vi "Handle Error in Client Generation.vi"(8 "error in":errorcluster) -> (0 "error out":errorcluster, 1 "InstrumentStudio Pro < Q4?":bool, 2 "status":T1, 3 "error message":string)   [LabVIEW 2021, in "MeasurementClient Editor.lvlib"]
uses:
  MeasurementClient Editor.lvlib
  Client Creation Status.ctl
  <vilib>/Utility/error.llb/DialogType.ctl
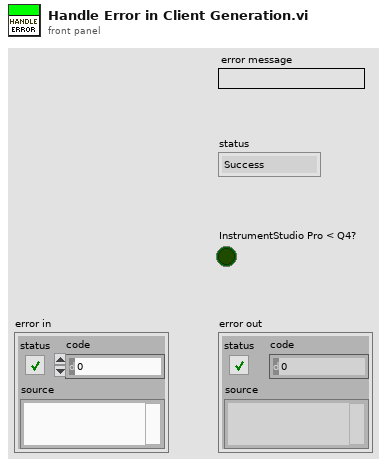
[diagram p1: front panel]
types:
  T1 = typedef "MeasurementClient Editor.lvlib/Client Creation Status.ctl" = enum16{"Success", "Fail"}
  T2 = typedef "DialogType.ctl" = u16
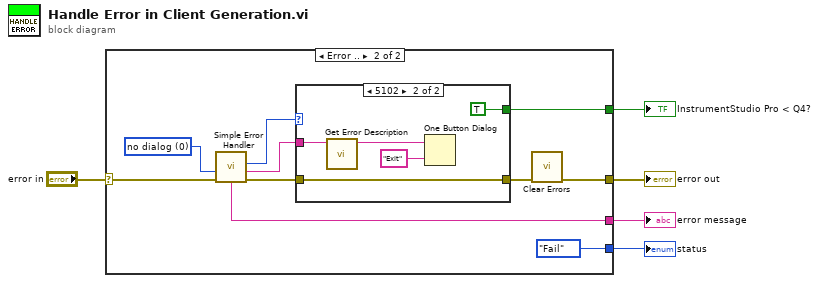
[diagram p0: block diagram]
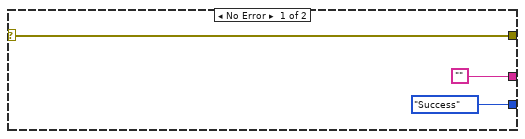
[diagram p2: hidden frame]
diagram:
  n1 = case shown="Error .." "error in" {
    selector: "error in" -> [w8 w18]
    tunnel: [w8 w17] -> w5
    tunnel: ["" w10] -> w3
    tunnel: [_ w12] -> w4
    tunnel: [Client_Creation_Status."Success" ("Enum") Client_Creation_Status."Fail" ("Enum")] -> w2
    frame No Error {
    }
    frame Error {
      w13 = T2 0 items=["no dialog", "OK message", "continue or stop message", "OK message + warnings", "continue/stop + warnings"] ("type of dialog (OK msg:1)")
      n2 = call <vilib>:"Simple Error Handler.vi"("type of dialog (OK msg:1)"=w13, "error in (no error)"=w18) -> ("code out"=w9:i32, "source out"=w14:string, "error out"=w16:errorcluster, "message"=w10:string)  [unwired: 3 in, 1 out]
      n3 = case shown="5102" w9 {
        tunnel: w16 -> [w19 w24]
        tunnel: [w19 w24] -> w15
        tunnel: w14 -> [_ w23]
        tunnel: [_ TRUE] -> w12
        frame 0, Default {
        }
        frame 5102 {
          n4 = call "Get Error Description.vi"("error source"=w23) -> ("error description"=w20:string)  [unwired: 10 in]
          n5 = One Button Dialog(message=w20, button name ("OK")="Exit") -> ()  [unwired: 1 out]
        }
      }
      n6 = call <vilib>:"Clear Errors.vi"("error in (no error)"=w15) -> ("error out"=w17:errorcluster)  [unwired: 5 in, 1 out]
    }
  }
  "error out" <- w5
  "error message" <- w3
  "InstrumentStudio Pro < Q4?" <- w4
  "status" <- w2
